vi "getTaskChannel.vi"(8 "error in (no error)":errorcluster, 11 "ITaskClassTemplate in":refnum<class "ITaskClassTemplate.lvclass">) -> (0 "error out":errorcluster, 2 "taskChannel":refnum<class "ITaskChannel.lvclass">, 3 "ITaskClassTemplate out":refnum<class "ITaskClassTemplate.lvclass">)   [LabVIEW 2023, in "ITaskClassTemplate.lvclass"]
doc: "Returns the Task Channel type used by the task."
uses:
  ITaskChannel/ITaskChannel.lvclass
  ITaskClassTemplate.lvclass
  ITaskClassTemplate.lvclass/ITaskClassTemplate.ctl
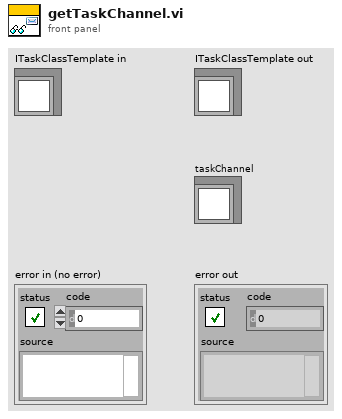
[diagram p1: front panel]
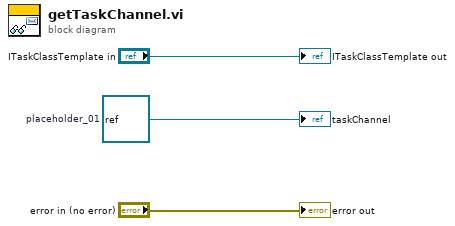
[diagram p0: block diagram]
diagram:
  w1 = refnum<class> refnum  # placeholder_01
  "error out" <- "error in (no error)"
  "ITaskClassTemplate out" <- "ITaskClassTemplate in"
  "taskChannel" <- w1
